vi "String - Parse String for Quotation Enclosed Text.vi"(8 "error in":errorcluster, 10 "Input String":string, 11 "Search String":string) -> (0 "error out":errorcluster, 3 "result string":string)   [LabVIEW 2020]
doc: "Search for a specified string, then return the value that follows & is contained within quotation marks.\nEg. for input string:\nip_addr: \"\\300\\250\\001\\001\"\nand search string:\nip_addr: \"\nThe returned value is:\n\\300\\250\\001\\001"
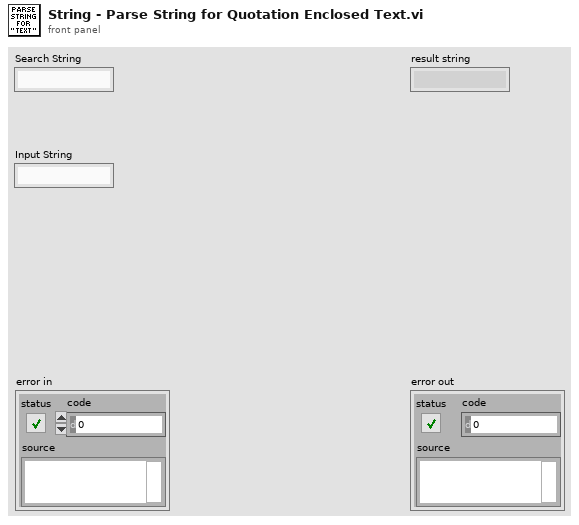
[diagram p1: front panel]
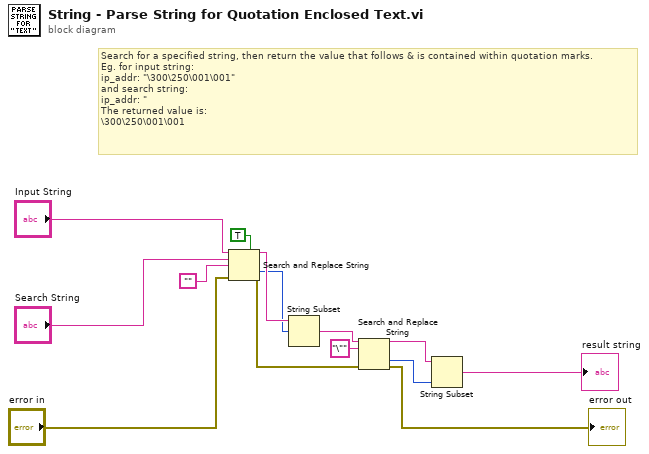
[diagram p0: block diagram]
diagram:
  # "Search for a specified string, then return the value that follows & is contained within quotation marks.\nEg. for input string:\nip_addr: \"\\300\\250\\001\\001\"\nand search string:\nip_addr: \"\nThe returned value is:\n\\300\\250\\001\\001"
  n1 = Search and Replace String(multiline?=TRUE ("multiline? (F)"), input string="Input String", search string="Search String", replace string="", error in="error in") -> (result string=w13:string, offset past replacement=w6:i32, error out=w2:errorcluster)  [unwired: 3 in, 1 out]
  n2 = String Subset(string=w13, offset (0)=w6) -> (substring=w7:string)  [unwired: 1 in]
  n3 = Search and Replace String(input string=w7, search string="\"", error in=w2) -> (result string=w9:string, offset past replacement=w10:i32, error out=→"error out":errorcluster)  [unwired: 5 in, 1 out]
  n4 = String Subset(string=w9, length (rest)=w10) -> (substring=→"result string":string)  [unwired: 1 in]
